vi "move to saved stage position.vi"(2 "error in":errorcluster, 3 "Stage VISA resource name in":refnum<visa-resource-name>, 4 "Position":i32, 5 "Saved Stage Positions":dbl[][](array[numeric])) -> (0 "VISA resource name out":refnum<visa-resource-name>, 1 "error out":errorcluster)   [LabVIEW 2016]
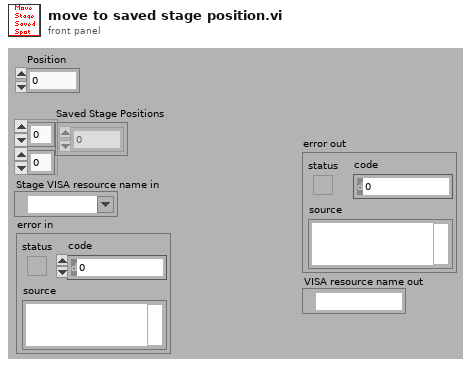
[diagram p1: front panel]
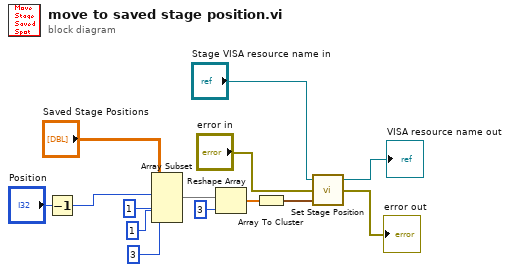
[diagram p0: block diagram]
diagram:
  n1 = Decrement(x="Position") -> (x-1=w1:i32)
  n2 = Array Subset(array="Saved Stage Positions", index (row)=w1, length (row)=1 ("length"), index (col)=1 ("index"), length (col)=3 ("length")) -> (w12:dbl[][])
  n3 = Reshape Array(w12, 3 ("dimension size")) -> (w10:dbl[])
  n4 = Array To Cluster(array=w10) -> (cluster=w8:cluster{"[0]":dbl, "[1]":dbl, "[2]":dbl})
  n5 = call "Set Stage Position.vi"("Position"=w8, "error in"="error in", "VISA resource name in"="Stage VISA resource name in") -> ("error out"=→"error out":errorcluster, "VISA resource name out"=→"VISA resource name out":refnum<visa-resource-name>)  [unwired: 1 out]
